vi "Get ODX Path.vi"(8 "error in (no error)":errorcluster, 11 "ODX type":string="File path") -> (0 "error out":errorcluster, 3 "Current Path":path)   [LabVIEW 2018]
uses:
  <vilib>/Utility/config.llb/Read Key (Path).vi
  <vilib>/Utility/config.llb/NI_LVConfig.lvlib
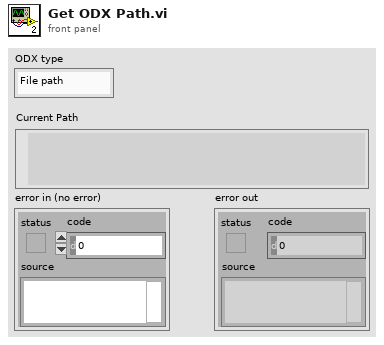
[diagram p1: front panel]
types:
  T1 = typedef "NI_LVConfig.lvlib/Config Data RefNum.ctl" = refnum<k1>
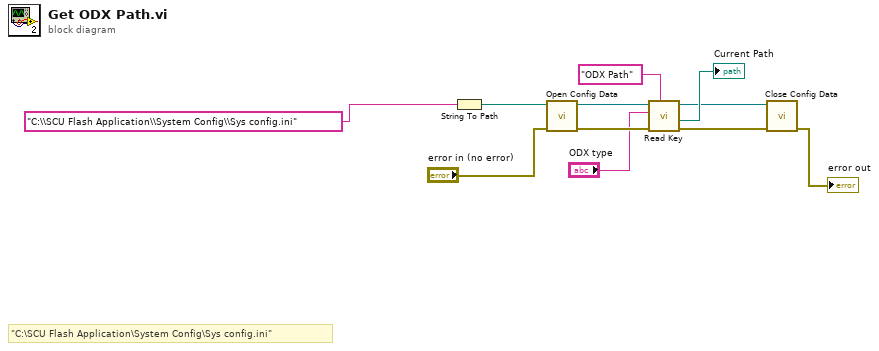
[diagram p0: block diagram]
diagram:
  # "\"C:\\SCU Flash Application\\System Config\\Sys config.ini\""
  n1 = String To Path(string="C:\\SCU Flash Application\\System Config\\Sys config.ini" ("name or relative path")) -> (path=w11:path)
  n2 = call <vilib>:"Open Config Data.vi"("error in (no error)"="error in (no error)", "configuration file path"=w11) -> ("error out"=w9:errorcluster, "refnum"=w10:T1)  [unwired: 7 in, 1 out]
  n3 = call-poly <vilib>:"Read Key.vi"("section"="ODX Path", "error in (no error)"=w9, "key"="ODX type", "refnum"=w10) -> ("error out"=w3:errorcluster, "value"=→"Current Path":path, "refnum out"=w4:T1)  [unwired: 4 in, 1 out]
  n4 = call <vilib>:"Close Config Data.vi"("error in (no error)"=w3, "refnum"=w4) -> ("error out"=→"error out":errorcluster)  [unwired: 8 in, 1 out]
